vi "Replace File Name.vi"(8 "error in (no error)":errorcluster, 10 "Actigraph ID":i32, 11 "File Ref In":refnum<file>) -> (0 "error out":errorcluster)   [LabVIEW 2017]
uses:
  Controls/control_all_in_one_package.ctl
  Controls/control_measurement_data.ctl
  Controls/control_measurement_settings.ctl
  Controls/control_memory_structure.ctl
  Controls/control_time_informations.ctl
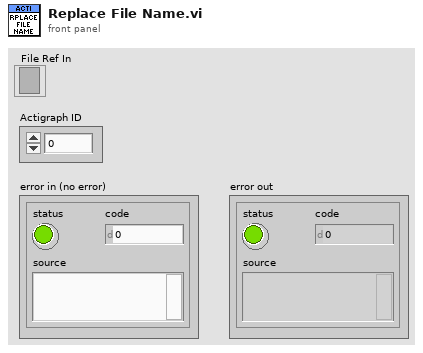
[diagram p1: front panel]
types:
  T1 = typedef "control_all_in_one_package.ctl" = cluster{"measurement data":T2, "actigraph settings":T3, "memory structure":T4, "time informations":T5}
  T2 = typedef "control_measurement_data.ctl" = cluster{"number of samples per axis":i32, "timestamp array":dbl[], "offset array":dbl[], "x, y, z axis data":waveform(dbl)[], "magnitude of acceleartion vectors":waveform(dbl), "statistics":cluster{"mean of x axis acceleration":dbl, "standard devation \nof x axis acceleration":dbl, "mean of y axis acceleration":dbl, "standard devation \nof y axis acceleration":dbl, "mean of z axis acceleration":dbl, "standard devation \nof z axis acceleration":dbl, "mean of magnitude\n of acceleration":dbl, "standard devation \nof magnitude of acceleration":dbl}, "voltage":waveform(dbl)}
  T3 = typedef "control_measurement_settings.ctl" = cluster{"sampling frequency [Hz]":dbl, "measurement interval [± g]":i32, "high precision?":bool, "number of pages":i32, "rate code":i32, "range code":i32, "id":i32}
  T4 = typedef "control_memory_structure.ctl" = cluster{"length of metadata [byte]":i32, "length of page [byte]":i32, "length of measurement \ndata on page [byte]":i32, "length of dataset [byte]":i32}
  T5 = typedef "control_time_informations.ctl" = cluster{"starting time":timestamp, "ending time":timestamp, "dt[s]":dbl, "sampling rate [Hz]":dbl, "length":dbl}
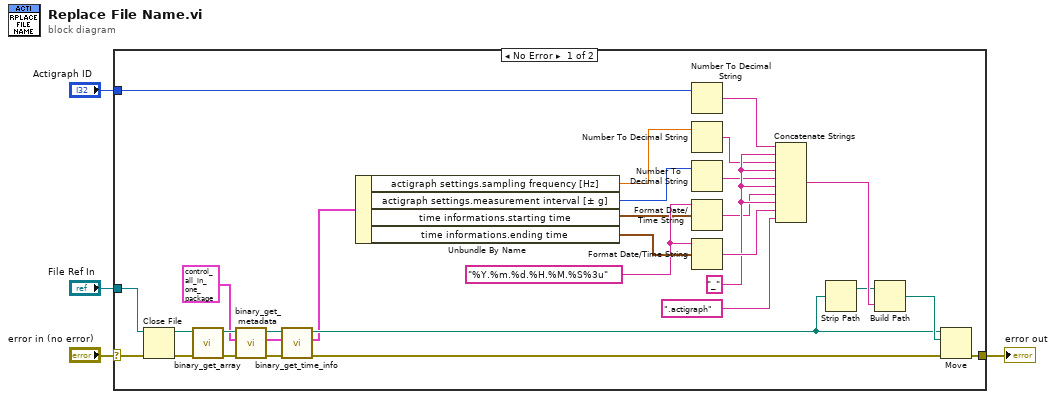
[diagram p0: block diagram]
diagram:
  n1 = case shown="No Error" "error in (no error)" {
    selector: "error in (no error)" -> [w6 w34]
    tunnel: "Actigraph ID" -> [w33 _]
    tunnel: [w28 w34] -> w3
    tunnel: "File Ref In" -> [w5 _]
    frame No Error {
      w24 = "_"
      w16 = "%Y.%m.%d.%H.%M.%S%3u" ("time format string (%c)")
      n2 = Close File(refnum=w5, error in=w6) -> (path=w29:path, error out=w7:errorcluster)
      n3 = call "binary_get_array.vi"("error in"=w7, "path to binary file"=w29) -> ("error out"=w9:errorcluster, "binary data"=w8:u8[])  [unwired: 8 in]
      n4 = call "binary_get_metadata.vi"("error in"=w9, "all in one package in"=T1 {"measurement data"={"number of samples per axis"=0, "timestamp array"=[], "offset array"=[], "x, y, z axis data"=[], "magnitude of acceleartion vectors"={"t0"=timestamp(0 s since 1904-01-01), "dt"=1.0, "Y"=[]}, "statistics"={"mean of x axis acceleration"=0.0, "standard devation \nof x axis acceleration"=0.0, "mean of y axis acceleration"=0.0, "standard devation \nof y axis acceleration"=0.0, "mean of z axis acceleration"=0.0, "standard devation \nof z axis acceleration"=0.0, "mean of magnitude\n of acceleration"=0.0, "standard devation \nof magnitude of acceleration"=0.0}, "voltage"={"t0"=timestamp(0 s since 1904-01-01), "dt"=1.0, "Y"=[]}}, "actigraph settings"={"sampling frequency [Hz]"=0.0, "measurement interval [± g]"=0, "high precision?"=FALSE, "number of pages"=0, "rate code"=0, "range code"=0, "id"=0}, "memory structure"={"length of metadata [byte]"=5, "length of page [byte]"=2048, "length of measurement \ndata on page [byte]"=2028, "length of dataset [byte]"=6}, "time informations"={"starting time"=timestamp(0 s since 1904-01-01), "ending time"=timestamp(0 s since 1904-01-01), "dt[s]"=0.0, "sampling rate [Hz]"=0.0, "length"=0.0}}, "binary data"=w8) -> ("error out"=w11:errorcluster, "all in one package out"=w13:T1, "pages"=w12:u8[])  [unwired: 6 in]
      n5 = call "binary_get_time_info.vi"("error in"=w11, "all in one package in"=w13, "pages"=w12) -> ("error out"=w27:errorcluster, "all in one package out"=w14:T1)  [unwired: 6 in, 1 out]
      n6 = Unbundle By Name(w14) -> ("actigraph settings.sampling frequency [Hz]"=w18:dbl, "actigraph settings.measurement interval [± g]"=w19:i32, "time informations.starting time"=w15:timestamp, "time informations.ending time"=w17:timestamp)
      n7 = Number To Decimal String(number=w33) -> (decimal integer string=w20:string)  [unwired: 1 in]
      n8 = Number To Decimal String(number=w18) -> (decimal integer string=w21:string)  [unwired: 1 in]
      n9 = Number To Decimal String(number=w19) -> (decimal integer string=w22:string)  [unwired: 1 in]
      n10 = Format Date/Time String(time format string (%c)=w16, seconds (now)=w15) -> (date/time string=w23:string)  [unwired: 1 in]
      n11 = Format Date/Time String(time format string (%c)=w16, seconds (now)=w17) -> (date/time string=w25:string)  [unwired: 1 in]
      n12 = Concatenate Strings(w20, w24, w21, w24, w22, w24, w23, w24, w25, ".actigraph") -> (w32:string)
      n13 = Strip Path(path=w29) -> (stripped path=w30:path)  [unwired: 1 out]
      n14 = Build Path(base path=w30, name or relative path=w32) -> (appended path=w31:path)
      n15 = Move(source path=w29, error in=w27, 10:w31) -> (error out=w28:errorcluster)  [unwired: 2 in, 2 out]
    }
    frame Error {
    }
  }
  "error out" <- w3
